vi "DeleteChannelConfirmation.vi"(8 "error in (no error)":errorcluster, 10 "Tag In":string) -> (0 "error out":errorcluster, 2 "Confirmed":bool)   [LabVIEW 2019]
panel:
  out "?":string
  in  "Btn-Cancel":bool
  in  "Btn-OK":bool
  # "Are you sure you want to delete this channel?"
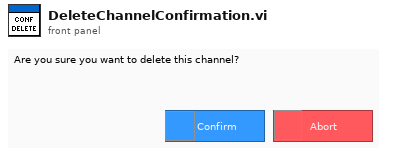
[diagram p1: front panel]
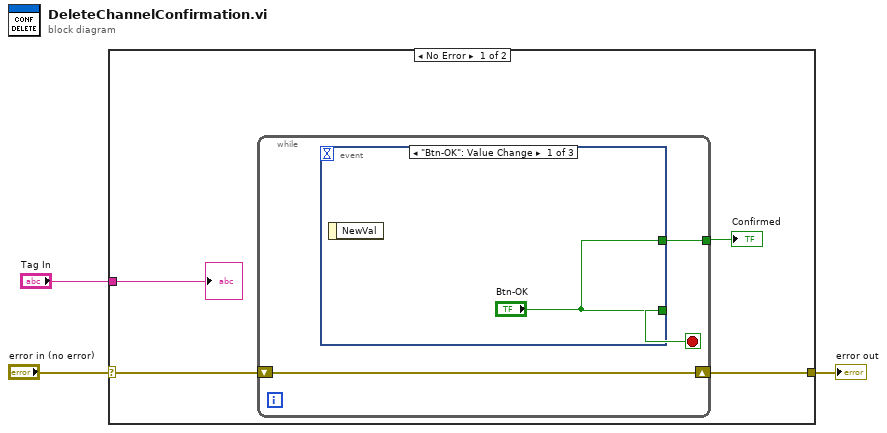
[diagram p0: block diagram]
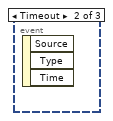
[diagram p2: hidden frame]
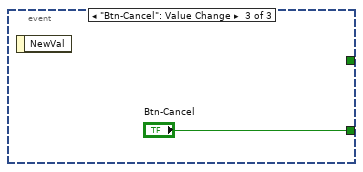
[diagram p3: hidden frame]
diagram:
  n1 = case shown="No Error" "error in (no error)" {
    selector: "error in (no error)" -> [w5 w13]
    tunnel: [w6 w13] -> w2
    tunnel: "Tag In" -> [w4 _]
    frame No Error {
      n2 = while {
        tunnel: [w9] -> w7
        shift-right: [w8] -> w6
        shift-left: w5 -> [w8]
        stop <- w10 stop-if-true
        n3 = event shown="[0] \"Btn-OK\": Value Change" {
          selector: _ -> [_ _ _]
          dyn-events: _ -> [_ _ _]
          timeout: _ -> [_ _ _]
          tunnel: ["Btn-OK" _ "Btn-Cancel"] -> w10
          tunnel: ["Btn-OK" _ _] -> w9
          event "Btn-OK": Value Change {
            n4 = event-data() -> ()  [unwired: 1 in, 1 out]
          }
          event Timeout {
            n5 = event-data() -> ()  [unwired: 1 in, 3 out]
          }
          event "Btn-Cancel": Value Change {
            n6 = event-data() -> ()  [unwired: 1 in, 1 out]
          }
        }
      }
      "Confirmed" <- w7
      "?" <- w4
    }
    frame Error {
    }
  }
  "error out" <- w2
